vi "ProcessingFrame.vi"(8 "error in (no error)":errorcluster, 11 "navX - Base in":refnum<class "navX - SERIAL.lvclass">) -> (0 "error out":errorcluster, 3 "navX - Base out":refnum<class "navX - SERIAL.lvclass">)   [LabVIEW 2015, in "navX Library v3.lvlib" / "navX - SERIAL.lvclass"]
uses:
  navX - SERIAL.lvclass
  navX - Interface/navX - Interface.lvclass
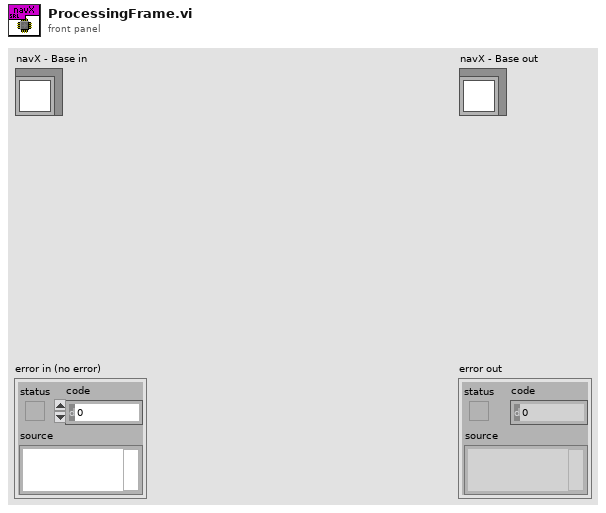
[diagram p1: front panel]
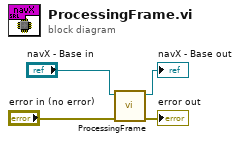
[diagram p0: block diagram]
diagram:
  n1 = call-parent "ProcessingFrame.vi"("error in (no error)"="error in (no error)", "navX - Base in"="navX - Base in") -> ("error out"=→"error out":errorcluster, "navX - Base out"=→"navX - Base out":refnum<class "navX - SERIAL.lvclass">)  [unwired: 8 in]
